vi "MoveComplete Event Callback.vi"(4 "?":refnum<vi>, 5 "Event Data":cluster{"lChanID":i32}, 6 "Control Ref":refnum<k7>, 7 "Event Common Data":T1) -> ()   [LabVIEW 2010]
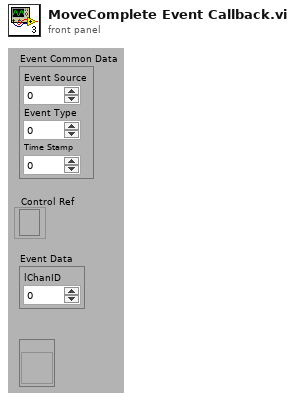
[diagram p1: front panel]
types:
  T1 = cluster{"Event Source":i32, "Event Type":u32, "Time Stamp":u32}
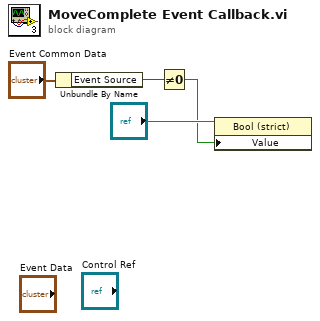
[diagram p0: block diagram]
diagram:
  n1 = Unbundle By Name("Event Common Data") -> ("Event Source"=w1:i32)
  n2 = Not Equal To 0?(x=w1) -> (x != 0?=w2:bool)
  n3 = property class="Bool (strict)"(reference="?", "Value"=w2) -> ()  [unwired: 1 in, 2 out]
